vi "Actor Core.vi"(8 "error in":errorcluster, 11 "CS++GoBangServer in":refnum<class "CS++GoBangServer.lvclass">) -> (0 "error out":errorcluster, 3 "Actor out":refnum<class "Actor.lvclass">)   [LabVIEW 2014, in "GoBang.lvlib" / "CS++GoBangServer.lvclass"]
doc: "(<B>Filename</B>: Actor Framework.lvlib:Actor.lvclass:Actor Core.vi)\n\nReceives messages to the actor, reacts to them, and initiates any error handling that may shut the actor down.\n\nDescendant classes may override this VI to append parallel tasks for the actor to complete while it handles messages. Overrides use the Call Parent Method node."
uses:
  CS++GoBangServer.lvclass
  <vilib>/ActorFramework/Actor/Actor.lvclass
  <vilib>/NI/Actors/Linked Network Actor/Linked Network Actor/Linked Network Actor.lvclass
  CS++GoBangServer.lvclass/CS++GoBangServer.ctl
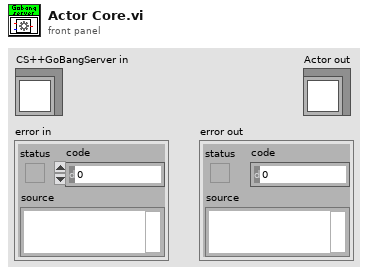
[diagram p1: front panel]
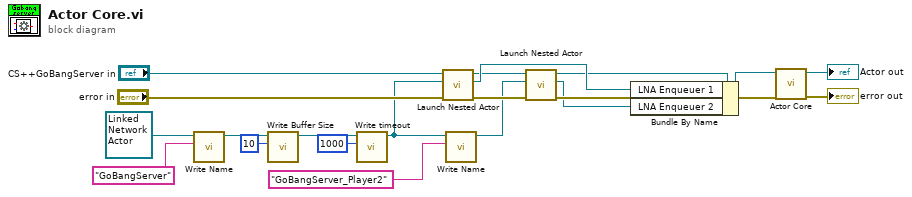
[diagram p0: block diagram]
diagram:
  n1 = call <vilib>:"Write Name.vi"("Name"="GoBangServer", "Network Actor in"=refnum<class "Linked Network Actor.lvclass"> refnum ("Network Actor.lvlib:Network Actor.lvclass")) -> ("Network Actor out"=w13:refnum<class "Linked Network Actor.lvclass">)  [unwired: 9 in]
  n2 = call <vilib>:"Write Buffer Size.vi"("Buffer Size"=10, "Network Actor in"=w13) -> ("Network Actor out"=w14:refnum<class "Linked Network Actor.lvclass">)  [unwired: 9 in]
  n3 = call <vilib>:"Write timeout.vi"("timeout"=1000, "Network Actor in"=w14) -> ("Network Actor out"=w3:refnum<class "Linked Network Actor.lvclass">)  [unwired: 9 in]
  n4 = call <vilib>:"Launch Nested Actor.vi"("error in (no error)"="error in", "Nested Actor"=w3, "Caller Actor in"="CS++GoBangServer in") -> ("error out"=w6:errorcluster, "Nested Actor's Enqueuer"=w9:refnum<class "Message Enqueuer.lvclass">, "Caller Actor out"=w8:refnum<class "CS++GoBangServer.lvclass">)  [unwired: 6 in]
  n5 = call <vilib>:"Write Name.vi"("Name"="GoBangServer_Player2", "Network Actor in"=w3) -> ("Network Actor out"=w2:refnum<class "Linked Network Actor.lvclass">)  [unwired: 9 in]
  n6 = call <vilib>:"Launch Nested Actor.vi"("error in (no error)"=w6, "Nested Actor"=w2, "Caller Actor in"=w8) -> ("error out"=w5:errorcluster, "Nested Actor's Enqueuer"=w4:refnum<class "Message Enqueuer.lvclass">, "Caller Actor out"=w7:refnum<class "CS++GoBangServer.lvclass">)  [unwired: 6 in]
  n7 = Bundle By Name(cluster=w7, "LNA Enqueuer 1"=w9, "LNA Enqueuer 2"=w4) -> (w10:refnum<class "CS++GoBangServer.lvclass">)
  n8 = call-parent "Actor Core.vi"("error in"=w5, "Actor in"=w10) -> ("error out"=→"error out":errorcluster, "Actor out"=→"Actor out":refnum<class "Actor.lvclass">)  [unwired: 8 in]
